vi "EEG_2022_040_LabView_4.1.vi"() -> ()   [LabVIEW 2022 SP3]
panel:
  in  "stop":bool
  out "error out":errorcluster
  in  "error in (no error)":errorcluster
  out "String":string
  out "Boolean":bool
  out "Numeric":dbl
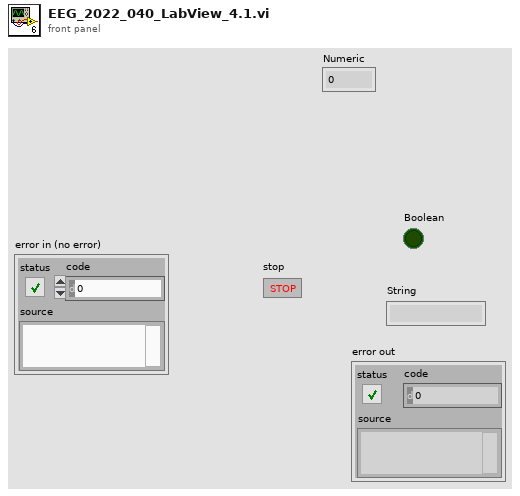
[diagram p1: front panel]
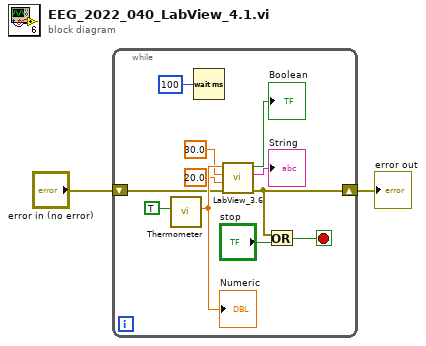
[diagram p0: block diagram]
diagram:
  n1 = while {
    shift-right: [w4] -> w1
    shift-left: "error in (no error)" -> [w6]
    stop <- w5 stop-if-true
    n2 = call "Thermometer.vi"("Temp Scale"=TRUE) -> ("Temperature"=w12:dbl)  [unwired: 9 in, 1 out]
    "Numeric" <- w12
    n3 = Wait (ms)(milliseconds to wait=100) -> ()  [unwired: 1 out]
    n4 = call "LabView_3.6.vi"("Error In"=w6, "Min.  Temperature"=20.0, "Max.  Temperature"=30.0, "Current  Temperatue"=w12) -> ("Error out"=w4:errorcluster, "Warning Text"=→"String":string, "Warning?"=→"Boolean":bool)  [unwired: 5 in]
    n5 = Or(x=w4, y="stop") -> (x .or. y?=w5:bool)
  }
  "error out" <- w1
